vi "PH_Trendviewer_Powermeter.evt Call Select Data.vi"(0 "i ref in":refnum<vi>, 1 "Stat or Trend":bool, 5 "error in (no error)":errorcluster, 6 "Instance":string="N/A") -> (14 "i ref out":refnum<vi>, 19 "error out":errorcluster)   [LabVIEW 2009, in "PH_Trendviewer_Powermeter.lvlib"]
doc: "This VI calls a certain ProcCase"
uses:
  PH_Trendviewer_Powermeter.lvlib
  CSCore/CSSystem/CoreLib/CoreLib.short 2 byte array.vi
  CSCore/BaseProcess/BaseProcess.lvlib
  CSCore/CSSystem/CoreLib/CoreLib.lvlib
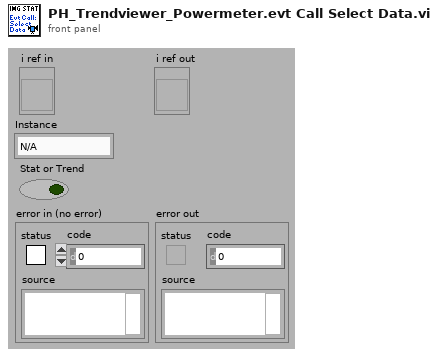
[diagram p1: front panel]
types:
  T1 = typedef "CoreDefs.rawDataType.ctl" = i8[]
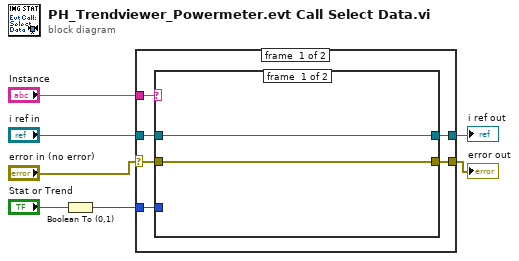
[diagram p0: block diagram]
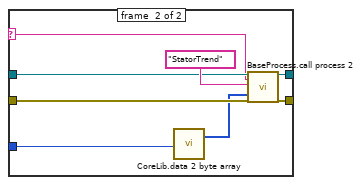
[diagram p2: hidden frame]
diagram:
  n1 = Boolean To (0,1)(Boolean="Stat or Trend") -> (0, 1=w1:i16)
  n2 = case shown="No Error" "error in (no error)" {
    selector: "error in (no error)" -> [w9 w24]
    tunnel: [w13 w25] -> w7
    tunnel: [w12 w24] -> w6
    tunnel: "i ref in" -> [w11 w25]
    tunnel: "Instance" -> [w10 _]
    tunnel: w1 -> [w8 _]
    frame #0 {
      n3 = case shown="Default" w10 {
        selector: w10 -> [_ w18]
        tunnel: [w15 w21] -> w13
        tunnel: [w14 w20] -> w12
        tunnel: w11 -> [w15 w19]
        tunnel: w9 -> [w14 w23]
        tunnel: w8 -> [_ w17]
        frame #0 {
        }
        frame #1 {
          n4 = call-poly "CoreLib.data 2 byte array.vi"("i16"=w17) -> ("byteArray out"=w16:T1)  [unwired: 18 in]
          n5 = call "BaseProcess.call process 2.vi"("i ref in"=w19, "Object"=w18, "Selector"="StatorTrend", "Data"=w16, "error in (no error)"=w23) -> ("i ref out"=w21:refnum<vi>, "error out"=w20:errorcluster)  [unwired: 13 in]
        }
      }
    }
    frame #1 {
    }
  }
  "error out" <- w6
  "i ref out" <- w7
